vi "NoLoopRunAndInitShiftregister.vi"() -> ()   [LabVIEW 2020]
panel:
  out "Numeric":i32
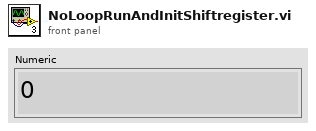
[diagram p1: front panel]
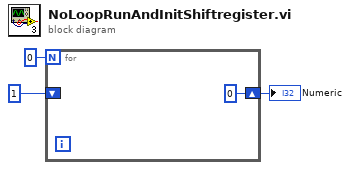
[diagram p0: block diagram]
diagram:
  n1 = for {
    N: 0 -> [_]
    shift-right: [0] -> w1
    shift-left: 1 -> [_]
  }
  "Numeric" <- w1
